vi "Item Select Menu.vi"(6 "State":T1, 9 "Index":i32, 11 "MenuRef":T10) -> ()   [LabVIEW 2020, in "FlexBlock.xnode"]
uses:
  FlexBlock.xnode
  <vilib>/XNodeSupport/XNodeMenuRef.ctl
  State.ctl
  FlexBlocks/Type Descriptor.ctl
  FlexBlocks/Terminal Direction.ctl
  FlexBlocks/Value Mode.ctl
  FlexBlocks/Terminal State.ctl
  FlexBlocks/Special Terminal.ctl
  FlexBlocks/Errors.ctl
  <vilib>/picture/picture.llb/imagedata.ctl
  FlexBlocks/Calculated Sizes.ctl
  FlexBlocks/Menu Action.ctl
  FlexBlocks/FlexBlocks.lvlib
  <vilib>/XNodeSupport/NI_XNodeSupport.lvlib
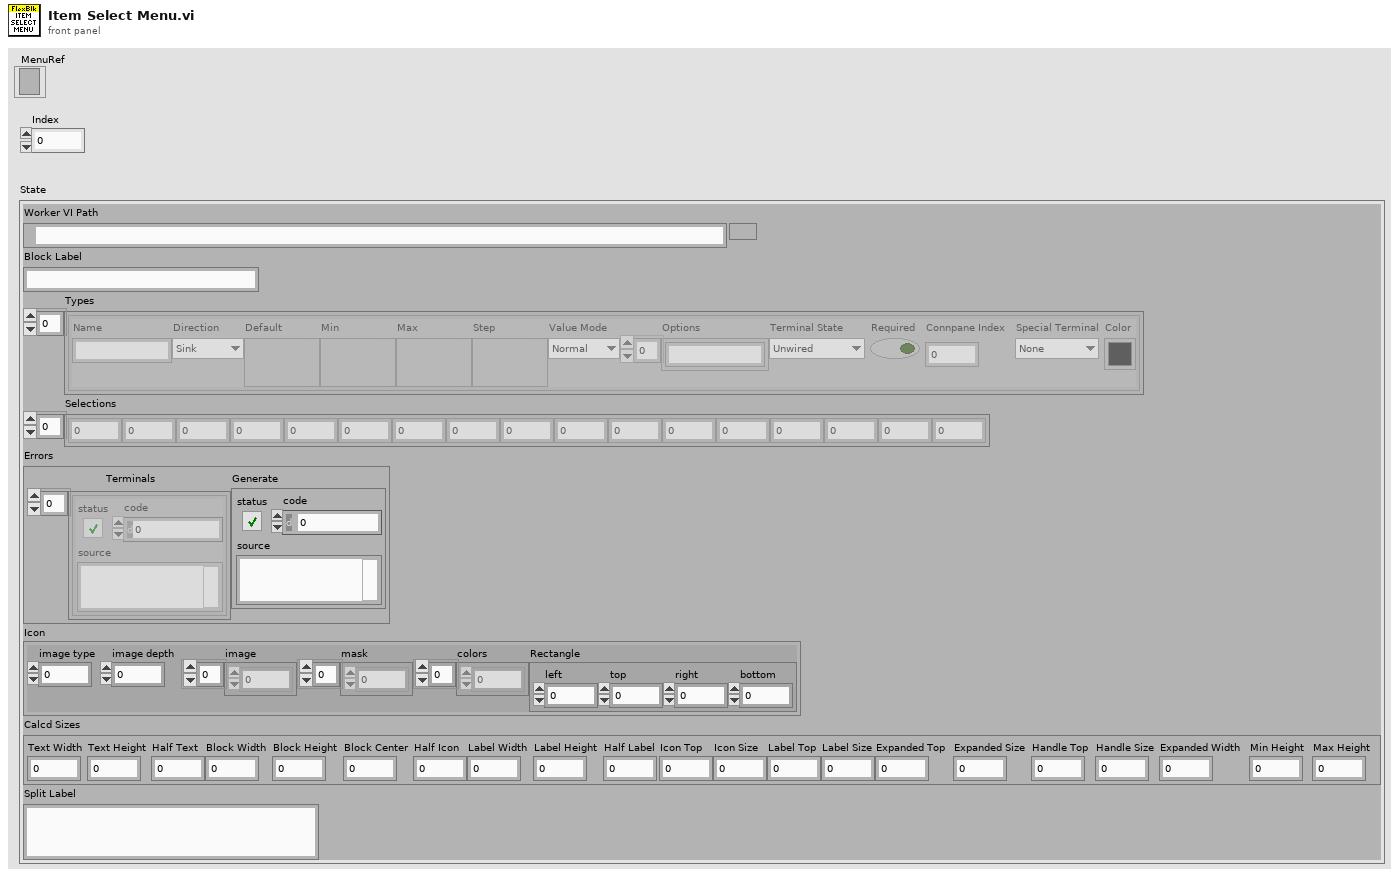
[diagram p1: front panel]
types:
  T1 = typedef "FlexBlock.xnode/State.ctl" = cluster{"Worker VI Path":path, "Block Label":string, "Types":T2[], "Selections":i32[], "Errors":T7, "Icon":T8, "Calcd Sizes":T9, "Split Label":string}
  T2 = typedef "FlexBlocks.lvlib/Type Descriptor.ctl" = cluster{"Name":string, "Direction":T3, "Default":variant, "Min":variant, "Max":variant, "Step":variant, "Value Mode":T4, "Options":string[], "Terminal State":T5, "Required":bool, "Connpane Index":i32, "Special Terminal":T6, "Color":u32}
  T3 = typedef "FlexBlocks.lvlib/Terminal Direction.ctl" = enum16{"Sink", "Source"}
  T4 = typedef "FlexBlocks.lvlib/Value Mode.ctl" = enum16{"Normal", "Range", "Select"}
  T5 = typedef "FlexBlocks.lvlib/Terminal State.ctl" = enum16{"Unwired", "BadType", "BadRef", "Channel", "Value", "Control Ref"}
  T6 = typedef "FlexBlocks.lvlib/Special Terminal.ctl" = enum16{"None", "Action", "Init", "Tag", "State in", "State out", "Error"}
  T7 = typedef "FlexBlocks.lvlib/Errors.ctl" = cluster{"Terminals":errorcluster[], "Generate":errorcluster}
  T8 = typedef "imagedata.ctl" = cluster{"image type":i32, "image depth":i32, "image":u8[], "mask":u8[], "colors":u32[], "Rectangle":cluster{"left":i16, "top":i16, "right":i16, "bottom":i16}}
  T9 = typedef "FlexBlocks.lvlib/Calculated Sizes.ctl" = cluster{"Text Width":i32, "Text Height":i32, "Half Text":i32, "Block Width":i32, "Block Height":i32, "Block Center":i32, "Half Icon":i32, "Label Width":i32, "Label Height":i32, "Half Label":i32, "Icon Top":i32, "Icon Size":i32, "Label Top":i32, "Label Size":i32, "Expanded Top":i32, "Expanded Size":i32, "Handle Top":i32, "Handle Size":i32, "Expanded Width":i32, "Min Height":i32, "Max Height":i32}
  T10 = typedef "NI_XNodeSupport.lvlib/XNodeMenuRef.ctl" = refnum<k9>
  T11 = typedef "FlexBlocks.lvlib/Menu Action.ctl" = enum16{"ITEM_SEL", "VAL_SEL"}
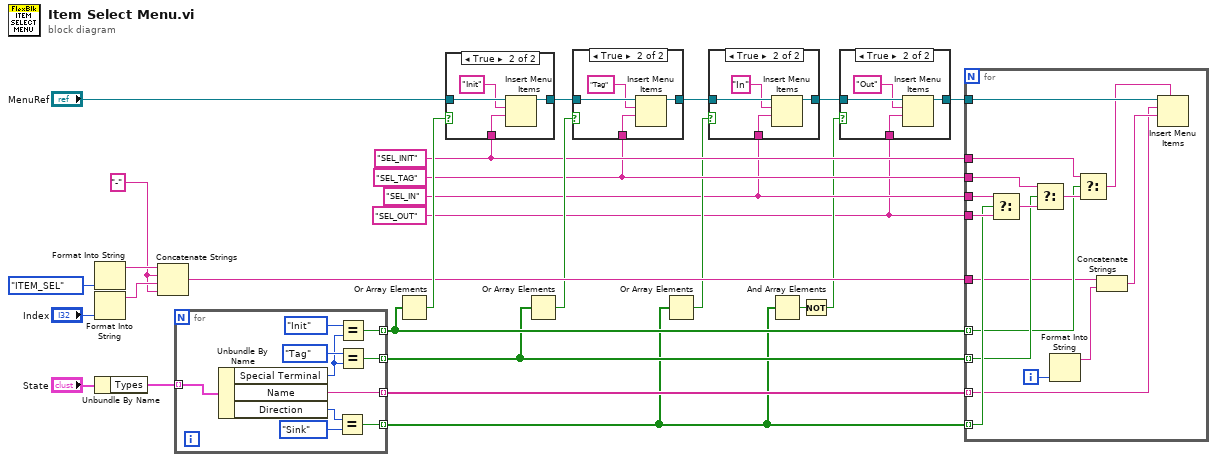
[diagram p0: block diagram]
diagram:
  w2 = "SEL_OUT"
  w7 = "SEL_IN"
  w10 = "SEL_TAG"
  w11 = "SEL_INIT"
  w20 = "-" ("string")
  n1 = Format Into String(Menu_Action."ITEM_SEL" ("Menu Action")) -> (resulting string=w22:string)  [unwired: 3 in, 1 out]
  n2 = Format Into String("Index") -> (resulting string=w21:string)  [unwired: 3 in, 1 out]
  n3 = Unbundle By Name("State") -> ("Types"=w25:T2[])
  n4 = Concatenate Strings(w22, w20, w21, w20) -> (w15:string)
  n5 = for {
    tunnel: w25 -> [w36] mode=indexing
    tunnel: [w32] -> w18 mode=indexing
    tunnel: [w31] -> w19 mode=indexing
    tunnel: [w28] -> w17 mode=indexing
    tunnel: [w27] -> w4 mode=indexing
    n6 = Unbundle By Name(w36) -> ("Special Terminal"=w33:T6, "Name"=w28:string, "Direction"=w30:T3)
    n7 = Equal?(x=w30, y=Terminal_Direction."Sink") -> (x = y?=w27:bool)
    n8 = Equal?(x=Special_Terminal."Init", y=w33) -> (x = y?=w31:bool)
    n9 = Equal?(x=Special_Terminal."Tag", y=w33) -> (x = y?=w32:bool)
  }
  n10 = Or Array Elements(Boolean array=w19) -> (logical OR=w16:bool)
  n11 = case shown="True" w16 {
    tunnel: "MenuRef" -> [w37 w41]
    tunnel: [w37 w39] -> w13
    tunnel: w11 -> [_ w38]
    frame False {
    }
    frame True {
      n12 = Insert Menu Items(7:w38, 8:"Init" ("item names"), 9:w41) -> (3:w39:refnum<k9>)  [unwired: 3 in, 2 out]
    }
  }
  n13 = Or Array Elements(Boolean array=w18) -> (logical OR=w12:bool)
  n14 = case shown="True" w12 {
    tunnel: w13 -> [w42 w46]
    tunnel: [w42 w44] -> w9
    tunnel: w10 -> [_ w43]
    frame False {
    }
    frame True {
      n15 = Insert Menu Items(7:w43, 8:"Tag" ("item names"), 9:w46) -> (3:w44:refnum<k9>)  [unwired: 3 in, 2 out]
    }
  }
  n16 = Or Array Elements(Boolean array=w4) -> (logical OR=w8:bool)
  n17 = case shown="True" w8 {
    tunnel: w9 -> [w47 w51]
    tunnel: [w47 w49] -> w6
    tunnel: w7 -> [_ w48]
    frame False {
    }
    frame True {
      n18 = Insert Menu Items(7:w48, 8:"In" ("item names"), 9:w51) -> (3:w49:refnum<k9>)  [unwired: 3 in, 2 out]
    }
  }
  n19 = And Array Elements(Boolean array=w4) -> (logical AND=w5:bool)
  n20 = Not(x=w5) -> (.not. x?=w3:bool)
  n21 = case shown="True" w3 {
    tunnel: w6 -> [w52 w56]
    tunnel: [w52 w54] -> w1
    tunnel: w2 -> [_ w53]
    frame False {
    }
    frame True {
      n22 = Insert Menu Items(7:w53, 8:"Out" ("item names"), 9:w56) -> (3:w54:refnum<k9>)  [unwired: 3 in, 2 out]
    }
  }
  n23 = for {
    tunnel: w19 -> [w64] mode=indexing
    tunnel: w18 -> [w67] mode=indexing
    tunnel: w4 -> [w70] mode=indexing
    tunnel: w17 -> [w57] mode=indexing
    tunnel: w15 -> [w60]
    tunnel: w11 -> [w65]
    tunnel: w10 -> [w68]
    tunnel: w7 -> [w72]
    tunnel: w2 -> [w71]
    tunnel: w1 -> [w63]
    i -> [w61]
    n24 = Select(t=w72, s=w70, f=w71) -> (s? t:f=w69:string)
    n25 = Select(t=w68, s=w67, f=w69) -> (s? t:f=w66:string)
    n26 = Format Into String(w61) -> (resulting string=w59:string)  [unwired: 3 in, 1 out]
    n27 = Select(t=w65, s=w64, f=w66) -> (s? t:f=w62:string)
    n28 = Concatenate Strings(w60, w59) -> (w58:string)
    n29 = Insert Menu Items(5:w62, 7:w58, 8:w57, 9:w63) -> ()  [unwired: 2 in, 3 out]
  }
